vi "API - Remove Rx Channels.vi"(8 "error in (no error)":errorcluster, 11 "Node Ptr":T1 format="%.0x") -> (0 "error out":errorcluster, 3 "Selected Channel Names":string[](array[string]))   [LabVIEW 2016, in "UDP-Custom-Device System Explorer.lvlib"]
uses:
  UDP-Custom-Device System Explorer.lvlib
  <vilib>/NI Veristand/Custom Device API/Custom Device Item Ref.ctl
  <vilib>/NI VeriStand/Custom Device API/Custom Device API.lvlib
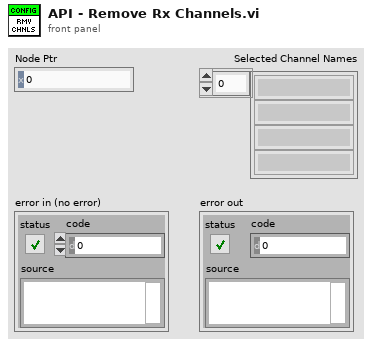
[diagram p1: front panel]
types:
  T1 = typedef "Custom Device API.lvlib/Custom Device Item Ref.ctl" = u64
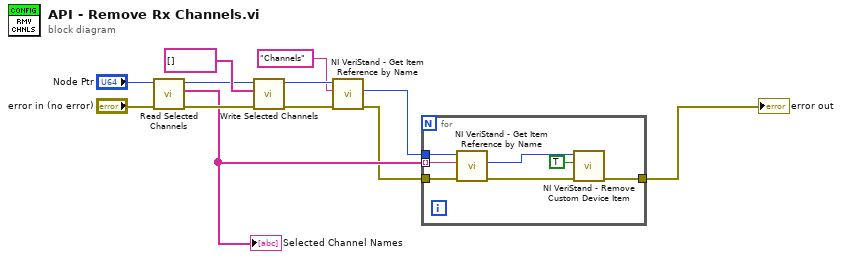
[diagram p0: block diagram]
diagram:
  n1 = call "Read Selected Channels.vi"("error in (no error)"="error in (no error)", "Node Ptr"="Node Ptr") -> ("error out"=w10:errorcluster, "Selected Channel Names"=w8:string[], "Node Ptr out"=w9:T1)  [unwired: 7 in]
  "Selected Channel Names" <- w8
  n2 = call "Write Selected Channels.vi"("error in (no error)"=w10, "Selected Channel Names"=string[] [] ("Selected Channel References"), "Node Ptr"=w9) -> ("error out"=w5:errorcluster, "Node Ptr out"=w3:T1)  [unwired: 7 in]
  n3 = call <vilib>:"NI VeriStand - Get Item Reference by Name.vi"("error in (no error)"=w5, "Item Name"="Channels" ("Numeric"), "Parent Ref in"=w3) -> ("error out"=w4:errorcluster, "Item Ref"=w2:T1)  [unwired: 5 in, 2 out]
  n4 = for {
    tunnel: w8 -> [w16] mode=indexing
    tunnel: w4 -> [w15]
    tunnel: [w19] -> w7
    tunnel: w2 -> [w17]
    n5 = call <vilib>:"NI VeriStand - Get Item Reference by Name.vi"("error in (no error)"=w15, "Item Name"=w16, "Parent Ref in"=w17) -> ("error out"=w13:errorcluster, "Item Ref"=w14:T1)  [unwired: 5 in, 2 out]
    n6 = call <vilib>:"NI VeriStand - Remove Custom Device Item.vi"("error in (no error)"=w13, "Force Delete (F)"=TRUE, "Item Ref in"=w14) -> ("error out"=w19:errorcluster)  [unwired: 7 in, 1 out]
  }
  "error out" <- w7
